vi "cRIO_4DoF_PluckerTrans.vi"(10 "Force control":dbl[](array[numeric]), 11 "d_{1}_{2} (mm)":dbl[](array[numeric])=[0.0, 0.0, 0.0]) -> (3 "TransF":dbl[](array[numeric]))   [LabVIEW 2019]
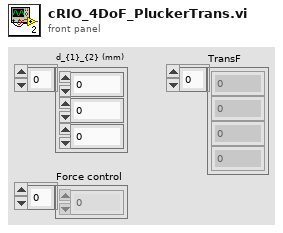
[diagram p1: front panel]
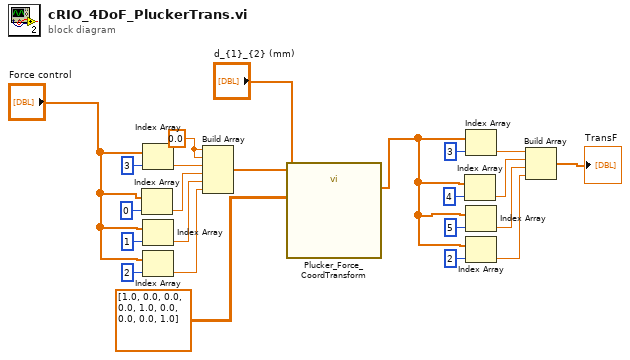
[diagram p0: block diagram]
diagram:
  w4 = 0.0 ("element")
  n1 = Index Array(array="Force control", index=0) -> (element=w8:dbl)
  n2 = Index Array(array="Force control", index=3) -> (element=w3:dbl)
  n3 = Index Array(array="Force control", index=1) -> (element=w9:dbl)
  n4 = Index Array(array="Force control", index=2) -> (element=w10:dbl)
  n5 = Build Array(w4, w4, w3, w8, w9, w10) -> (w11:dbl[])
  n6 = call "Plucker_Force_CoordTransform.vi"("R_{1}_{2}"=dbl[][] [[1.0, 0.0, 0.0], [0.0, 1.0, 0.0], [0.0, 0.0, 1.0]], "d_{1}_{2} (mm)"="d_{1}_{2} (mm)", "F_{1}"=w11) -> ("F_{2}"=w22:dbl[])  [unwired: 8 in]
  n7 = Index Array(array=w22, index=4) -> (element=w19:dbl)
  n8 = Index Array(array=w22, index=3) -> (element=w15:dbl)
  n9 = Index Array(array=w22, index=5) -> (element=w20:dbl)
  n10 = Index Array(array=w22, index=2) -> (element=w21:dbl)
  n11 = Build Array(w15, w19, w20, w21) -> (→"TransF":dbl[])
